vi "Get VIs with Debugging Disabled.vi"(8 "error in (no error)":errorcluster, 11 "Coverage Analyzer Result View in":refnum<class "Coverage Analyzer Result View.lvclass">) -> (0 "error out":errorcluster, 2 "VIs":set{path}(c389), 3 "Coverage Analyzer Result View out":refnum<class "Coverage Analyzer Result View.lvclass">)   [LabVIEW 2020, in "Coverage Analyzer Result View.lvclass"]
uses:
  Coverage Analyzer Result View.lvclass
  Coverage Analyzer Result View.lvclass/Coverage Analyzer Result View.ctl
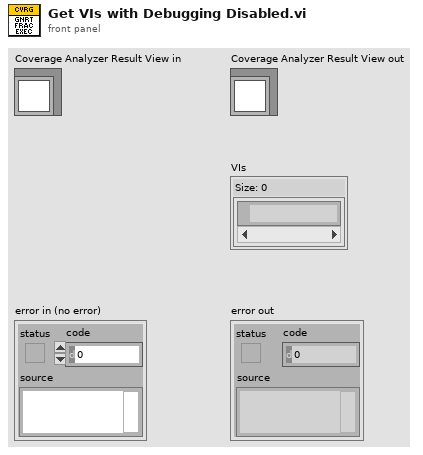
[diagram p1: front panel]
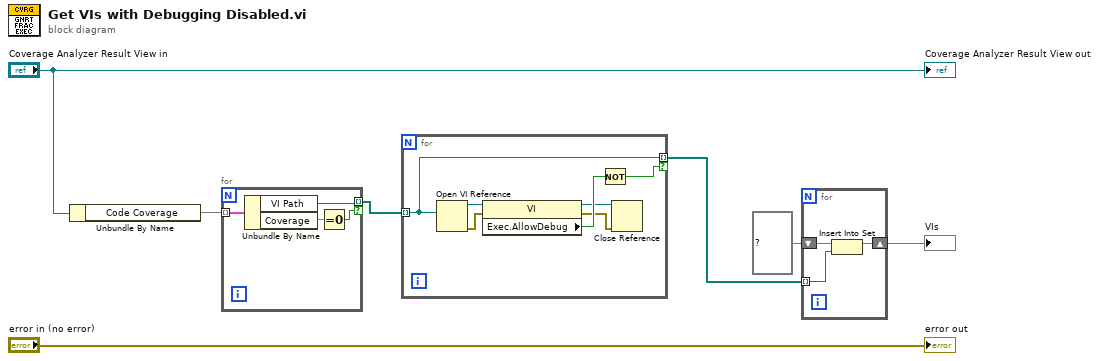
[diagram p0: block diagram]
diagram:
  n1 = Unbundle By Name("Coverage Analyzer Result View in") -> ("Code Coverage"=w2:map{path, dbl})
  n2 = for {
    tunnel: w2 -> [w11] mode=indexing
    tunnel: [w8] -> w7 mode=indexing if=w9
    n3 = Unbundle By Name(w11) -> ("VI Path"=w8:path, "Coverage"=w10:dbl)
    n4 = Equal To 0?(x=w10) -> (x = 0?=w9:bool)
  }
  n5 = for {
    tunnel: w7 -> [w13] mode=indexing
    tunnel: [w13] -> w4 mode=indexing if=w12
    n6 = Open VI Reference(vi path=w13) -> (vi reference=w18:refnum<vi>, error out=w17:errorcluster)  [unwired: 5 in]
    n7 = property class="VI"(reference=w18, error in=w17) -> (reference out=w14:refnum<vi>, error out=w15:errorcluster, "Exec.AllowDebug"=w16:bool)
    n8 = Not(x=w16) -> (.not. x?=w12:bool)
    n9 = Close Reference(reference=w14, error in (no error)=w15) -> ()  [unwired: 1 out]
  }
  n10 = for {
    shift-right: [w20] -> w6
    shift-left: set{path} {} ("VIs") -> [w21]
    tunnel: w4 -> [w19] mode=indexing
    n11 = Insert Into Set(10:w19, 11:w21) -> (3:w20:set{path})  [unwired: 1 out]
  }
  "VIs" <- w6
  "error out" <- "error in (no error)"
  "Coverage Analyzer Result View out" <- "Coverage Analyzer Result View in"
